vi "ExSubCloseFileImageMulti.vi"(1 "error in (no error)":errorcluster, 2 "Handles In":T1) -> (0 "error out":errorcluster)   [LabVIEW 2013]
panel:
  # "ExSubCloseFileImage:\nThis is a subVI which takes a cluster of handles and closes the file, and image only"
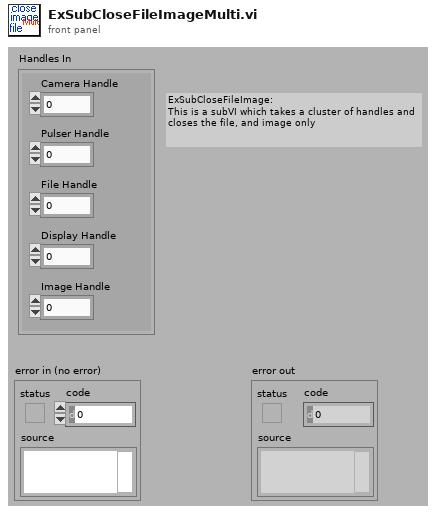
[diagram p1: front panel]
types:
  T1 = cluster{"Camera Handle":u32, "Pulser Handle":u32, "File Handle":u32, "Display Handle":u32, "Image Handle":u32}
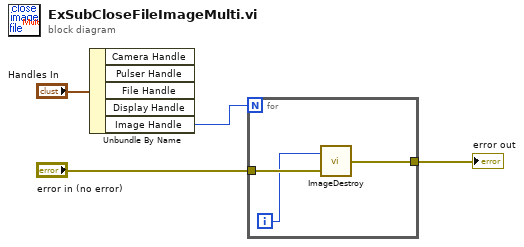
[diagram p0: block diagram]
diagram:
  n1 = Unbundle By Name("Handles In") -> ("Image Handle"=w1:u32)  [unwired: 4 out]
  n2 = for {
    N: w1 -> [_]
    tunnel: [w7] -> w3
    tunnel: "error in (no error)" -> [w6]
    i -> [w5]
    n3 = call <userlib>:"ImageDestroy.vi"("error in"=w6, "Data handle"=w5) -> ("error out"=w7:errorcluster)
  }
  "error out" <- w3
